vi "Bind I32 parameter.vi"(4 "error in (no error)":errorcluster, 6 "Parameter":i32, 7 "Statement Refnum":T1) -> (0 "error out":errorcluster, 3 "Statement Refnum":T1)   [LabVIEW 2011]
doc: "Charge le paramètre de type enier long (I32) dans la pile"
uses:
  SQL Controls/Statement Refnum.ctl
  Odbc32.dll
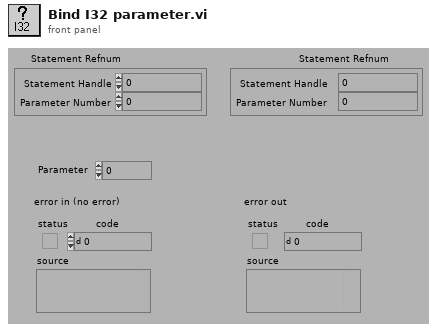
[diagram p1: front panel]
types:
  T1 = typedef "Statement Refnum.ctl" = cluster{"Statement Handle":i32, "Parameter Number":u16}
  T2 = enum16{"NOPE", "SQL_HANDLE_ENV", "SQL_HANDLE_DBC", "SQL_HANDLE_STMT", "SQL_HANDLE_DESC"}
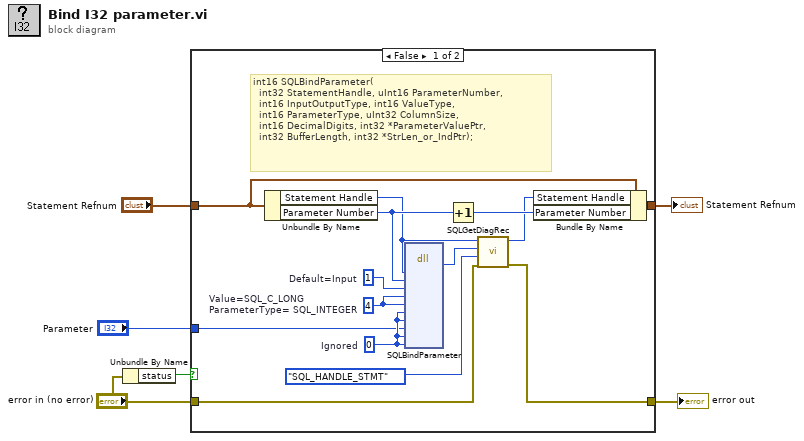
[diagram p0: block diagram]
diagram:
  n1 = Unbundle By Name("error in (no error)") -> ("status"=w2:bool)
  n2 = case shown="False" w2 {
    tunnel: "Statement Refnum" -> [w20 w22]
    tunnel: [w19 w22] -> w5
    tunnel: "error in (no error)" -> [w13 w21]
    tunnel: [w9 w21] -> w3
    tunnel: "Parameter" -> [w8 _]
    frame False {
      w14 = i16 4  # Value=SQL_C_LONG ParameterType= SQL_INTEGER
      w15 = 0  # Ignored
      w17 = i16 1  # Default=Input
      # "int16 SQLBindParameter(\n  int32 StatementHandle, uInt16 ParameterNumber, \n  int16 InputOutputType, int16 ValueType, \n  int16 ParameterType, uInt32 ColumnSize, \n  int16 DecimalDigits, int32 *ParameterValuePtr,\n  int32 BufferLength, int32 *StrLen_or_IndPtr);"
      n3 = Unbundle By Name(w20) -> ("Statement Handle"=w12:i32, "Parameter Number"=w18:u16)
      n4 = dll-call lib="Odbc32.dll" fn="SQLBindParameter"("StatementHandle"=w12, "ParameterNumber"=w18, "InputOutputType"=w17, "ValueType"=w14, "ParameterType"=w14, "ColumnSize"=w15, "DecimalDigits"=w15, "ParameterValuePtr"=w8, "BufferLength"=w15, "StrLen_or_IndPtr"=w15) -> (w10:i16)  [unwired: 11 in, 4 out]
      n5 = Increment(x=w18) -> (x+1=w16:u16)
      n6 = call "SQLGetDiagRec.vi"("error in (no error)"=w13, "HandleType"=T2."SQL_HANDLE_STMT", "Status (SQL_SUCCESS=0)"=w10, "Input Handle"=w12) -> ("error out"=w9:errorcluster, "Output Handle"=w11:i32)  [unwired: 2 out]
      n7 = Bundle By Name(cluster=w20, "Statement Handle"=w11, "Parameter Number"=w16) -> (w19:T1)
    }
    frame True {
    }
  }
  "Statement Refnum" <- w5
  "error out" <- w3
